vi "HELLO WORLD.vi"() -> ()   [LabVIEW 2019]
panel:
  out "STRING":string
  # "HELLO WORLD"
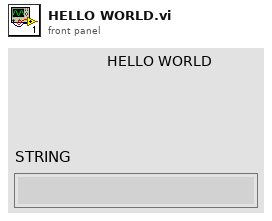
[diagram p1: front panel]
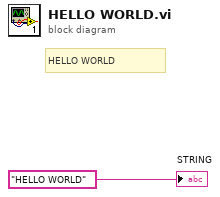
[diagram p0: block diagram]
diagram:
  # "HELLO WORLD"
  "STRING" <- "HELLO WORLD" ("STRING")
